vi "One-Click Deployment.vi"() -> ()   [LabVIEW 2012]
uses:
  <vilib>/AppBuilder/AB_API_Simple/Build (path).vi
  <vilib>/regexp/Match Regular Expression.xnode
  <vilib>/AppBuilder/AB_API_Simple/NI_App_Builder_API.lvlib
  Deployment/Deployment Support/AWS-S3-MiniAPI.lvclass
panel:
  out "Tab Control":T1(tab)
  out "CurrentStep":string
  in  "Setup Script":string="[Setup]\nAppName=Finite Measurement Demo\nAppVersion=1.0.0.2\nDefaultDirName={pf}\\\\Finite Measurement Demo\nAppId=Finite Measurement Demo\nAppContact=\"Jack Dunaway\" <jack@wirebirdlabs.com>\nAppPublisher=Wirebird Labs LLC\nAppPublisherURL=https://wirebirdlabs.com\nAppSupportPhone=512-981-LABS\nAppSupportURL=https://connect.wirebirdlabs.com\nAppCopyright=Copyright © 2012-2013 Wirebird Labs LLC.\nOutputDir=%s\nOutputBaseFilename=Finite Measurement Installer\nDisableDirPage=yes\nDisableProgramGroupPage=yes\nWizardImageFile=DefaultSideBanner.bmp\nWizardSmallImageFile=DefaultTopImage.bmp\n\n[Components]\n; Name: \"LV2012_RTE\"; Description: \"Install LabVIEW Run-Time Engine\"\n\n[Files]\nSource: \"%s\\\\*\"; DestDir: \"{app}\"; Flags: recursesubdirs\nSource: \"%s\\\\*\"; DestDir: \"{tmp}\\\\InstallLabVIEWRTE\"; Flags: recursesubdirs deleteafterinstall\n\n[Messages]\n;FinishedLabelNoIcons=Let's get rolling!\n\n[Run]\nFilename: msiexec.exe; Parameters: \"/i \"\"{tmp}\\\\InstallLabVIEWRTE\\\\LV2012runtime.msi\"\" /quiet /norestart\"; WorkingDir: {tmp}; StatusMsg: \"Installing LabVIEW Run-Time Engine...\"\n; Filename: msiexec.exe; Parameters: \"/i \"\"{tmp}\\\\InstallLabVIEWRTE\\\\mkl.msi\"\" /quiet /norestart\"; WorkingDir: {tmp}; StatusMsg: \"Installing LabVIEW Math Kernel Libraries...\"\nFilename: \"{app}\\\\Main.exe\"; Description: \"Launch Finite Measurement Demo\"; Flags: postinstall nowait skipifsilent\n\n\n\n\n\n"
  in  "Download Page HTML":string="\n<!DOCTYPE HTML>\n<html dir=\"ltr\" lang=\"en-US\">\n\n<head>\n\n\t<!-- Title -->\n\t<title>CLA Summit 2013</title>\n\t\n\t<!-- SEO -->\n\t<meta name=\"robots\" content=\"noindex,noarchive,nosnippet\" />\n\n\t<!-- Stylesheets -->\n \t<link rel=\"stylesheet\" type=\"text/css\" media=\"all\" href=\"http://deploy.wirebirdlabs.com/Resources/Bootstrap/css/bootstrap.min.css\" />\n\t<link rel=\"stylesheet\" type=\"text/css\" media=\"all\" href=\"http://deploy.wirebirdlabs.com/Resources/FontAwesome/css/font-awesome.min.css\" />\n\t<link rel=\"stylesheet\" type=\"text/css\" media=\"all\" href=\"http://deploy.wirebirdlabs.com/Resources/Themes/Default/style.css\" />\n\n\t<!-- Scripts -->\n \t<script type='text/javascript' src='https://ajax.googleapis.com/ajax/libs/jquery/1.8.2/jquery.min.js'></script>\n\t<script type='text/javascript' src='http://deploy.wirebirdlabs.com/Resources/Bootstrap/js/bootstrap.min.js'></script>\n\n</head>\n\n<body class=\"container page-background\">\n\n\t<div class=\"container page-canvas\">\n\t\t<div class=\"page-header\">\n\t\t\t<h1 class=\"page-title page-title-title\">CLA Summit 2013:<br>Deployment Automation Demo</h1>\n\t\t</div>\n\n\t\t<div class=\"page-body\">\n\n\t\t\t<div class=\"row page-top-block\">\n\t\t\t\t\t\t\t<div class=\"row page-top-block\">\n\t\t\t\t<div class=\"span7 offset1 app-intro-block\">\n\t\t\t\t\t<h1 class=\"page-title page-title-featured-release\">Latest Release</h1>\n\t\t\t\t\t<h5>This application is a demo for the American CLA Summit 2013.</h5>\n\t\t\t\t\t<div class=\"featured-changes\">\n\t\t\t\t\t\t<table class=\"changelog-list table table-striped subtle-shadow\">\n\t\t\t\t\t\t\t<thead>\n\t\t\t\t\t\t\t\t<tr><th colspan=\"2\">Finite Measurement Demo<span class=\"release-date\">04 Mar 2013</span></th></tr>\n\t\t\t\t\t\t\t</thead>\n\t\t\t\t\t\t\t<tbody>\n\t\t\t\t\t\t\t\t<tr><td class=\"change-feature\">Bugfix</td><td>Feature request #455 is implemented.</td></tr>\n\t\t\t\t\t\t\t\t<tr><td class=\"change-bugfix\">Bugfix</td><td>Bug report #456 is resolved</td></tr>\n\t\t\t\t\t\t\t</tbody>\n\t\t\t\t\t\t</table>\n\n\t\t\t\t\t</div>\n\t\t\t\t\t<a href=\"http://demo.wirebirdlabs.com/Installer.exe\" class=\"download-link btn btn-large btn-success\">\n       Download Installer<span class=\"download-size\">32.5MB</span>\n     </a>\n\t\t\t\t</div>\n\n\t\t\t\t<div class=\"contact-block span3\">\n\t\t\t\t\t<h1 class=\"contact-heading\">Support</h1>\n\t\t\t\t\t<p class=\"contact-name\">Jack Dunaway</p>\n\t\t\t\t\t<p class=\"contact-email\">support@wirebirdlabs.com</p>\n\t\t\t\t\t<p class=\"contact-phone\">512-981-LABS</p>\n\t\t\t\t\t<p class=\"contact-hours\">9AM-9PM CST</p>\n\t\t\t\t\t<p class=\"contact-website\"><a href=\"https://connect.wirebirdlabs.com\" target=\"_blank\">Technical Support Website</a></p>\n\t\t\t\t\t<a class=\"documentation-link btn btn-info\" href=\"https://connect.wirebirdlabs.com/knowledgebase/topics/22620\" target=\"_blank\">Documentation</a>\n\t\t\t\t</div>\n\t\t\t</div>\n\t\t</div>\n\n<div class=\"row accordion changelog-block\"></div>\n\n\t\t<div class=\"page-footer row-fluid\">\n\t\t\t<span class=\"span12\"></span>\n\t\t</div>\n  </div>\n\t</div>\n\n\t<footer class=\"\">\n\n\t\t<p class=\"page-copyright\">Copyright &copy; 2013 Wirebird Labs LLC.</p>\n\n\t\t<!-- Bootstrap Scripts -->\n\t\t<script type='text/javascript'>\n\t\t\tjQuery(document).ready( function(){\n\t\t\t\tjQuery('*[rel=popover]').popover();\n\t\t\t\tjQuery('*[rel=tooltip]').tooltip();} );\n\t\t</script>\n\t</footer>\n</body>\n</html>"
  in  "Access Key":string="AKIAIHIOPAOX2ODZ6J3Q"
  in  "Secret Key":string
  in  "S3 Bucket":string="demo.wirebirdlabs.com"
  out "Installer Filepath":string
  out "ResponseXml":string
  out "Object Download URL":string
  out "Inno Error":string
  out "error out":errorcluster
  out "Inno Output":string
  # "Jack Dunaway - CLA - LabVIEW Champion"
  # "Jack Dunaway - CLA - LabVIEW Champion"
  # "Deployment Automation and\nRelease Engineering for LabVIEW"
  # "Deployment Automation and\nRelease Engineering for LabVIEW"
  # "Follow along:"
  # "Follow along:"
  # "join.me/wirebirdlabs"
  # "join.me/wirebirdlabs"
  # "Download code:"
  # "Download code:"
  # "wirebird.co/CLA-Summit-2013-Austin"
  # "wirebird.co/CLA-Summit-2013-Austin"
  # "1. A Basic One-Click Deployment Automation Script\n\n2. Automating Inno Setup from the Command Line\n\n3. Uploading Application Installers to the web\n\n4. Creating a human-friendly Download Page for your customers\n\n5. Segmenting the Run-Time Engine and Dependencies for smaller installer footprint\n\n6. Use of Virgin Virtual Machines and Snapshots to test Deployments and End-User Experience\n\n7. You can open the webpage on your own computer and install this application!!"
  # "1. A Basic One-Click Deployment Automation Script\n\n2. Automating Inno Setup from the Command Line\n\n3. Uploading Application Installers to the web\n\n4. Creating a human-friendly Download Page for your customers\n\n5. Segmenting the Run-Time Engine and Dependencies for smaller installer footprint\n\n6. Use of Virgin Virtual Machines and Snapshots to test Deployments and End-User Experience\n\n7. You can open the webpage on your own computer and install this application!!"
  # "Agenda"
  # "Agenda"
  # "... the Ideal DevX:\nThe One-click deployment\n\n... the Ideal Customer Experience:\nThe Forehead Install"
  # "... the Ideal DevX:\nThe One-click deployment\n\n... the Ideal Customer Experience:\nThe Forehead Install"
  # "Goal: To approximate, or even achieve..."
  # "Goal: To approximate, or even achieve..."
  # "Inno Setup, free, open source setup authoring:\nhttp://www.jrsoftware.org/isinfo.php\n\nAmazon AWS SDK for .NET\nhttp://aws.amazon.com/sdkfornet/\n\nSegment the Run-Time Engine to minimize installer footprint:\nhttp://wirebird.co/Minify-RTE\n\nWirebird Labs Deploy: polished, powerful deployment automation\nhttps://wirebirdlabs.com/deploy"
  # "Inno Setup, free, open source setup authoring:\nhttp://www.jrsoftware.org/isinfo.php\n\nAmazon AWS SDK for .NET\nhttp://aws.amazon.com/sdkfornet/\n\nSegment the Run-Time Engine to minimize installer footprint:\nhttp://wirebird.co/Minify-RTE\n\nWirebird Labs Deploy: polished, powerful deployment automation\nhttps://wirebirdlabs.com/deploy"
  # "Links"
  # "Links"
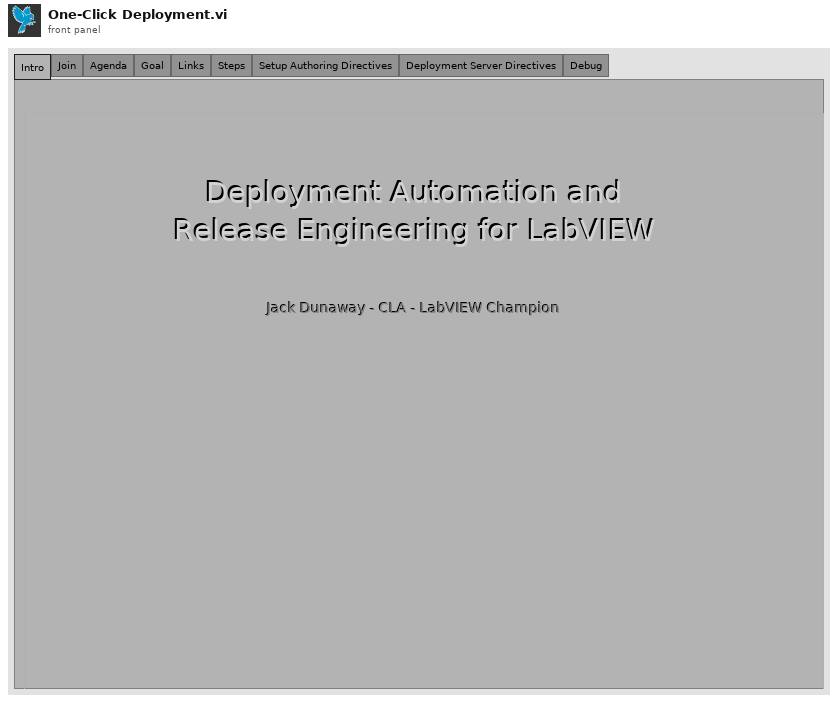
[diagram p1: front panel]
types:
  T1 = enum32{"Intro", "Join", "Agenda", "Goal", "Links", "Steps", "Setup Authoring Directives", "Deployment Server Directives", "Debug"}
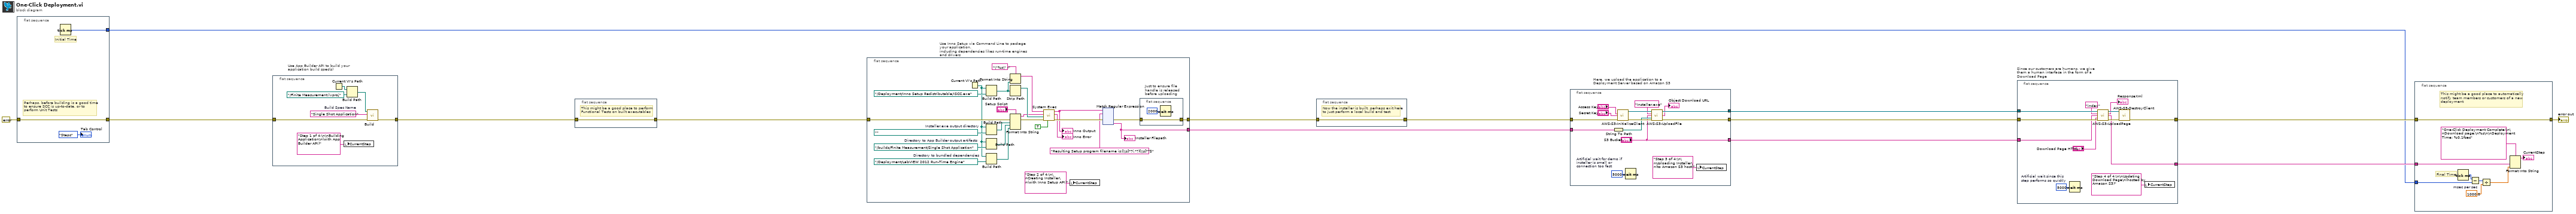
[diagram p0: block diagram]
diagram:
  n1 = flat-sequence {
    tunnel: [w17] -> w6
    tunnel: errorcluster {"status"=FALSE, "code"=0, "source"=""} ("error in (no error)") -> [w17]
    tunnel: [w16] -> w3
    frame #0 {
      # "Initial Time"
      # "Perhaps, before building is a good time\nto ensure SCC is up-to-date, or to\nperform Unit Tests"
      n2 = Tick Count (ms)() -> (millisecond timer value=w16:u32)
      "Tab Control" <- T1."Steps" ("Tab Control")
    }
  }
  n3 = flat-sequence "Use App Builder API to build your\napplication build spec(s)" {
    tunnel: [w20] -> w9
    tunnel: w6 -> [w19]
    frame #0 {
      w24 = "Single Shot Application"  # Build Spec Name
      n4 = Current VI's Path() -> (path=w23:path)
      n5 = local write "CurrentStep"("Step 1 of 4:\n\nBuilding Application\n(with App Builder API)" ("CurrentStep")) -> ()
      n6 = Build Path(base path=w23, name or relative path=path "../Finite Measurement.lvproj" ("Path to project")) -> (appended path=w21:path)
      n7 = call-poly <vilib>:"Build.vi"("error in (no error)"=w19, "Name of build specification (if empty: build all)"=w24, "Path to project"=w21) -> ("error out"=w20:errorcluster)  [unwired: 7 in, 1 out]
    }
  }
  n8 = flat-sequence {
    tunnel: [w25] -> w10
    tunnel: w9 -> [w25]
    frame #0 {
      # "This might be a good place to perform\nFunctional Tests on built executables"
    }
  }
  n9 = flat-sequence "Use Inno Setup via Command Line to package your application,\nincluding dependencies likes run-time engines and drivers" {
    tunnel: [w44] -> w14
    tunnel: w10 -> [w35]
    tunnel: [w29] -> w2
    frame #0 {
      w33 = path ".."  # Installer.exe output directory
      w38 = path "../Deployment/LabVIEW 2012 Run-Time Engine"  # Directory to bundled dependencies
      w39 = path "../builds/Finite Measurement/Single Shot Application"  # Directory to App Builder output artifacts
      n10 = Current VI's Path() -> (path=w32:path)
      n11 = Build Path(base path=w32, name or relative path=path "../Deployment/Inno Setup Redistributable/ISCC.exe" ("Path to project")) -> (appended path=w48:path)
      n12 = Build Path(base path=w32, name or relative path=w33) -> (appended path=w34:path)
      n13 = Build Path(base path=w32, name or relative path=w39) -> (appended path=w40:path)
      n14 = Build Path(base path=w32, name or relative path=w38) -> (appended path=w37:path)
      n15 = Format Into String(format string="\"%s\" -", w48) -> (resulting string=w46:string)  [unwired: 2 in, 1 out]
      n16 = Strip Path(path=w48) -> (stripped path=w47:path)  [unwired: 1 out]
      n17 = Format Into String(format string="Setup Script", error in=w35, w34, w40, w37) -> (resulting string=w41:string, error out=w36:errorcluster)  [unwired: 1 in]
      n18 = call <vilib>:"System Exec.vi"("run minimized? (F)"=TRUE, "error in (no error)"=w36, "working directory"=w47, "standard input"=w41, "command line"=w46) -> ("error out"=w45:errorcluster, "standard error"=→"Inno Error":string, "standard output"=w28:string)  [unwired: 3 in, 1 out]
      "Inno Output" <- w28
      n19 = local write "CurrentStep"("Step 2 of 4:\n\nCreating Installer\n(with Inno Setup API)" ("CurrentStep")) -> ()
      n20 = xnode "Match Regular Expression"("input string"=w28, "regular expression"="Resulting Setup program filename is:[\\s]*?(.*?)[\\s]*?$", "error in"=w45) -> ("error out"=w30:errorcluster, "submatch 1"=w44:string)  [unwired: 3 in, 4 out]
      "Installer Filepath" <- w44
      n21 = flat-sequence "Just to ensure file\nhandle is released\nbefore uploading" {
        tunnel: w30 -> [w51]
        tunnel: [w51] -> w29
        frame #0 {
          n22 = Wait (ms)(milliseconds to wait=u32 2000) -> ()  [unwired: 1 out]
        }
      }
    }
  }
  n23 = flat-sequence {
    tunnel: [w166] -> w1
    tunnel: w2 -> [w166]
    frame #0 {
      # "Now the installer is built, perhaps exit here\nto just perform a local build and test"
    }
  }
  n24 = flat-sequence "Here, we upload the application to a\nDeployment Server based on Amazon S3" {
    tunnel: w14 -> [w180]
    tunnel: [w176] -> w13
    tunnel: [w175] -> w12
    tunnel: ["S3 Bucket"] -> w11
    tunnel: w1 -> [w170]
    frame #0 {
      w167 = u32 5000  # Artificial wait for demo if installer is small or connection too fast
      n25 = String To Path(string=w180) -> (path=w177:path)
      n26 = call "AWS-S3-InitializeClient.vi"("Access Key"="Access Key", "Secret Key"="Secret Key", "error in"=w170) -> ("Mini AWS S3 API"=w178:refnum<class "AWS-S3-MiniAPI.lvclass">, "error out"=w179:errorcluster)  [unwired: 11 in]
      n27 = Wait (ms)(milliseconds to wait=w167) -> ()  [unwired: 1 out]
      n28 = call "AWS-S3-UploadFile.vi"("Mini AWS S3 API"=w178, "Object Key"="Installer.exe", "Object Bucket"="S3 Bucket", "Source Filepath (Local)"=w177, "error in"=w179) -> ("Mini AWS S3 API out"=w176:refnum<class "AWS-S3-MiniAPI.lvclass">, "Object Download URL"=→"Object Download URL":string, "error out"=w175:errorcluster)  [unwired: 8 in]
      n29 = local write "CurrentStep"("Step 3 of 4:\n\nUploading Installer\n(to Amazon S3 host)" ("CurrentStep")) -> ()
    }
  }
  n30 = flat-sequence "Since our customers are humans, we give\nthem a human interface in the form of a Download Page" {
    tunnel: [w192] -> w8
    tunnel: w13 -> [w191]
    tunnel: w12 -> [w190]
    tunnel: w11 -> [w183]
    tunnel: [w182] -> w4
    frame #0 {
      w181 = u32 5000  # Artificial wait since this step performs so quickly
      n31 = Wait (ms)(milliseconds to wait=w181) -> ()  [unwired: 1 out]
      n32 = call "AWS-S3-UploadPage.vi"("Mini AWS S3 API"=w191, "Object Key"="index", "Object Bucket"=w183, "Object Data"="Download Page HTML", "error in"=w190) -> ("Mini AWS S3 API out"=w188:refnum<class "AWS-S3-MiniAPI.lvclass">, "ResponseXml"=→"ResponseXml":string, "Download Page URL"=w182:string, "error out"=w187:errorcluster)  [unwired: 7 in]
      n33 = call "AWS-S3-DestroyClient.vi"("Mini AWS S3 API"=w188, "error in"=w187) -> ("error out"=w192:errorcluster)  [unwired: 13 in]
      n34 = local write "CurrentStep"("Step 4 of 4:\n\nUpdating Download Page\n(hosted by Amazon S3)" ("CurrentStep")) -> ()
    }
  }
  n35 = flat-sequence {
    tunnel: [w201] -> w7
    tunnel: w8 -> [w201]
    tunnel: w4 -> [w194]
    tunnel: w3 -> [w199]
    frame #0 {
      w197 = 1000.0  # msec per sec
      # "Final Time"
      # "This might be a good place to automatically\nnotify team members or customers of a new\ndeployment"
      n36 = Tick Count (ms)() -> (millisecond timer value=w200:u32)
      n37 = Subtract(x=w200, y=w199) -> (x-y=w198:u32)
      n38 = Divide(x=w198, y=w197) -> (x/y=w193:dbl)
      n39 = Format Into String(format string="One-Click Deployment Complete!\n\nDownload page:\n%s\n\nDeployment Time: %0.1fsec" ("CurrentStep"), w194, w193) -> (resulting string=→"CurrentStep":string)  [unwired: 2 in, 1 out]
    }
  }
  "error out" <- w7
